vi "HFRR ADV v017 new software.vi"() -> ()   [LabVIEW 2025] (continued)
                n3041 = call <vilib>:"Write Characters To File.vi"("append to file? (new file:F)"=FALSE, "character string"=w3783, "file path (dialog if empty)"=w3788) -> ()  [unwired: 2 in, 1 out]
              }
            }
          }
          frame Enabled {
          }
        }
        n3042 = case shown="True" "OK Button 17" {
          frame False {
          }
          frame True {
            (unwired) 0  # existing file
            w4041 = "Choose a datalog file to open"  # prompt
            n3043 = local write "OK Button 17"(FALSE ("OK Button 17")) -> ()
            n3044 = local read "String"() -> (w4036:string)
            n3045 = String To Path(string=w4036) -> (path=w4037:path)
            n3046 = File Dialog(6:"*.duf" ("pattern"), 7:w4041, 11:w4037) -> (0:w4028:errorcluster, 3:w4047:path)  [unwired: 4 in, 2 out]
            n3047 = Unbundle(w4028) -> ()  [unwired: 3 out]
            n3048 = Open/Create/Replace File "Open File"(file path (use dialog)=w4047) -> (refnum out=w4039:refnum<file>)  [unwired: 5 in, 2 out]
            n3049 = Strip Path(path=w4047) -> (name=w4045:string)  [unwired: 1 out]
            n3050 = Path To String(path=w4047) -> (string=w4030:string)
            n3051 = while {
              tunnel: w4039 -> [w4051]
              i -> [w4048]
              stop <- w4049 continue-if-true
              (unwired) TRUE ("line mode (F)")
              n3052 = Read from Text File "Read File"(file (use dialog)=w4051) -> (text=w4050:string)  [unwired: 3 in, 3 out]
              n3053 = local write "Numeric 16"(w4048) -> ()
              n3054 = String Length(string=w4050) -> (length=w4053:i32)
              n3055 = Greater?(x=w4053, y=1) -> (0:w4049:bool)
            }
            n3056 = local write "String 29"(w4030) -> ()
            n3057 = Search and Replace String(input string=w4030, search string=".duf", replace string=".dgf" ("replace string (\"\")")) -> (result string=→"String Indicator 4":string)  [unwired: 5 in, 3 out]
            n3058 = Match Pattern(string=w4045, regular expression=".dwm") -> (before substring=w4029:string)  [unwired: 1 in, 3 out]
            "String Indicator" <- w4029
            n3059 = Match Pattern(string=w4030, regular expression=".dwm" ("substring (\"\")")) -> (before substring=w4031:string)  [unwired: 1 in, 3 out]
            "String Indicator 3" <- w4031
            n3060 = local write "TITTLE 2"(w4029) -> ()
            n3061 = String To Path(string=w4031) -> (path=w4038:path)
            "path" <- w4038
            n3062 = call <vilib>:"Read Characters From File.vi"("file path (dialog if empty)"=w4038, "start of read offset (chars.:0)"=60 ("start of read offset (chars.: 0)")) -> ("character string"=→"String Indicator 2":string)  [unwired: 4 in, 3 out]
          }
        }
        n3063 = call <vilib>:"Query Available Printers.vi"() -> ("system configured printers"=w3730:string[])  [unwired: 9 in, 2 out]
        "System Configured Printers 2" <- w3730
        n3064 = local read "OK Button 16"() -> (w3727:bool)
        n3065 = case shown="True" "OK Button 16" {
          frame False {
          }
          frame True {
            n3066 = stacked-sequence {
              frame #0 {
                n3067 = local read "Numeric 16"() -> (w4055:i32)
                n3068 = local write "Numeric 10"(w4055) -> ()
              }
              frame #1 {
                n3069 = local read "S.NO"() -> (→"s.NO":string)
                n3070 = local read "String 29"() -> (w4059:string)
                n3071 = String To Path(string=w4059) -> (path=w4058:path)
                n3072 = Open/Create/Replace File "Open File"(file path (use dialog)=w4058) -> (refnum out=w4060:refnum<file>)  [unwired: 5 in, 2 out]
                n3073 = for {
                  N: 16 -> [_]
                  tunnel: w4060 -> [w4067]
                  i -> [w4063]
                  (unwired) TRUE ("line mode (F)")
                  n3074 = Read from Text File "Read File"(file (use dialog)=w4067) -> (text=w4061:string)  [unwired: 3 in, 3 out]
                  n3075 = Match Pattern(string=w4061, regular expression="(") -> (after substring=w4066:string)  [unwired: 1 in, 3 out]
                  n3076 = Match Pattern(string=w4066, regular expression=")") -> (before substring=w4062:string)  [unwired: 1 in, 3 out]
                  n3077 = case shown="1" w4063 {
                    tunnel: w4062 -> [w4068 w4069 _ _ w4070 w4071 w4072 w4074 w4076 w4078 w4080 w4082 w4084 w4086 _]
                    tunnel: w4061 -> [_ _ _ _ _ _ _ _ _ _ _ _ _ _ _]
                    frame 0 {
                      "TITTLE" <- w4068
                    }
                    frame 1 {
                      "Sample ID" <- w4069
                    }
                    frame 2 {
                    }
                    frame 3 {
                    }
                    frame 4 {
                      "Test Date" <- w4070
                    }
                    frame 5 {
                      "Tested by" <- w4071
                    }
                    frame 6 {
                      n3078 = Fract/Exp String To Number(string=w4072) -> (number=→"Humidity before test 2":dbl)  [unwired: 3 in, 1 out]
                    }
                    frame 7 {
                      n3079 = Fract/Exp String To Number(string=w4074) -> (number=→"Temperature before test 2":dbl)  [unwired: 3 in, 1 out]
                    }
                    frame 8 {
                      n3080 = Fract/Exp String To Number(string=w4076) -> (number=→"Humidity after test 2":dbl)  [unwired: 3 in, 1 out]
                    }
                    frame 9 {
                      n3081 = Fract/Exp String To Number(string=w4078) -> (number=→"Temperature after test 2":dbl)  [unwired: 3 in, 1 out]
                    }
                    frame 10 {
                      n3082 = Fract/Exp String To Number(string=w4080) -> (number=→"MWSD 2":dbl)  [unwired: 3 in, 1 out]
                    }
                    frame 11 {
                      n3083 = Fract/Exp String To Number(string=w4082) -> (number=→"AVP 2":dbl)  [unwired: 3 in, 1 out]
                    }
                    frame 12 {
                      n3084 = Fract/Exp String To Number(string=w4084) -> (number=→"HCF 2":dbl)  [unwired: 3 in, 1 out]
                    }
                    frame 13 {
                      n3085 = Fract/Exp String To Number(string=w4086) -> (number=→"WS1.4 2":dbl)  [unwired: 3 in, 1 out]
                    }
                    frame 14, Default {
                    }
                  }
                }
              }
              frame #2 {
              }
            }
            n3086 = local write "OK Button 16"(FALSE ("OK Button 13")) -> ()
          }
        }
        n3087 = Index Array(array=w3730, index="Select Printer 3") -> (element=w3732:string)
        "Selected Printer" <- w3732
        n3088 = case shown="True" w3727 {
          frame False {
          }
          frame True {
            n3089 = flat-sequence {
              frame #0 {
              }
              frame #1 {
                n3090 = Wait (ms)(milliseconds to wait=u32 100) -> ()  [unwired: 1 out]
              }
              frame #2 {
                n3091 = local write "OK Button 16"(FALSE ("Print 3")) -> ()
              }
            }
          }
        }
        n3092 = case shown="True" "Print" {
          tunnel: w3732 -> [_ w4024]
          frame False {
          }
          frame True {
            (unwired) i16 6 ("width (-)")
            (unwired) "TESTED BY : "
            (unwired) "TESTED DATE :"
            (unwired) "SAMPLE ID : "
            (unwired) "SAMPLE DESIGN : "
            w3982 = "\r"
            w3999 = "\r"
            # "add image"
            n3093 = local read "Sample ID"() -> (w3972:string)
            n3094 = local read "Tested by"() -> (w3975:string)
            n3095 = local read "String 34"() -> (w3962:string)
            n3096 = local read "String 45"() -> (w3942:string)
            n3097 = local read "String 35"() -> (w3957:string)
            n3098 = local read "String 37"() -> (w3955:string)
            n3099 = local read "String 32"() -> (w3977:string)
            n3100 = local read "String 36"() -> (w3952:string)
            n3101 = local read "String 31"() -> (w3976:string)
            n3102 = local read "Test Date"() -> (w3973:string)
            n3103 = local read "String 33"() -> (w3978:string)
            n3104 = local read "String 38"() -> (w3948:string)
            n3105 = local read "String 39"() -> (w3945:string)
            n3106 = local write "Print"(FALSE ("Print FF")) -> ()
            n3107 = local read "S 39"() -> (w3960:string)
            n3108 = local read "S 38"() -> (w3967:string)
            n3109 = local read "Temperature before test 2"() -> (w3998:dbl)
            n3110 = local read "Temperature after test 2"() -> (w3988:dbl)
            n3111 = local read "Humidity before test 2"() -> (w4013:dbl)
            n3112 = local read "Humidity after test 2"() -> (w3997:dbl)
            n3113 = local read "MWSD 2"() -> (w4002:dbl)
            n3114 = local read "WS1.4 2"() -> (w3980:dbl)
            n3115 = Concatenate Strings("2)" ("string"), w3962) -> (w3963:string)
            n3116 = Concatenate Strings("3)" ("string"), w3960) -> (w3961:string)
            n3117 = Concatenate Strings("1)" ("string"), w3967) -> (w3966:string)
            n3118 = Concatenate Strings("4)" ("string"), w3957) -> (w3958:string)
            n3119 = Concatenate Strings("5)" ("string"), w3955) -> (w3954:string)
            n3120 = Concatenate Strings("6)" ("string"), w3952) -> (w3951:string)
            n3121 = Concatenate Strings("7)" ("string"), w3948) -> (w3949:string)
            n3122 = Concatenate Strings("8)" ("string"), w3945) -> (w3946:string)
            n3123 = local read "HCF 2"() -> (w3984:dbl)
            n3124 = local read "AVP 2"() -> (w4001:dbl)
            n3125 = local read "s.NO"() -> (w3943:string)
            n3126 = call <vilib>:"New Report.vi"("report type"=enum16{"Standard Report", "HTML"}."Standard Report") -> ("report out"=w4022:refnum<class "NI_report.lvclass">, "error out"=w4021:errorcluster)  [unwired: 13 in]
            n3127 = local read "TITTLE"() -> (w3974:string)
            n3128 = Concatenate Strings(w3999, w3942, w3943, w3999, w3977, w3972, w3999, w3976, w3973, w3999, w3978, w3975, w3999) -> (w3992:string)
            "test by" <- w3992
            n3129 = Number To Fractional String(number=w3998, width (-)=i16 6, precision (6)=i16 2) -> (F-format string=w3987:string)  [unwired: 1 in]
            n3130 = Number To Fractional String(number=w3997, width (-)=i16 6, precision (6)=i16 2) -> (F-format string=w4000:string)  [unwired: 1 in]
            n3131 = Number To Fractional String(number=w4013, width (-)=i16 6, precision (6)=i16 2) -> (F-format string=w4018:string)  [unwired: 1 in]
            n3132 = Number To Fractional String(number=w4002, width (-)=i16 6, precision (6)=i16 2) -> (F-format string=w4004:string)  [unwired: 1 in]
            n3133 = Number To Fractional String(number=w3988, width (-)=i16 6, precision (6)=i16 2) -> (F-format string=w3989:string)  [unwired: 1 in]
            n3134 = Number To Fractional String(number=w4001, width (-)=i16 6, precision (6)=i16 2) -> (F-format string=w4003:string)  [unwired: 1 in]
            n3135 = Number To Fractional String(number=w3984, width (-)=i16 6, precision (6)=i16 2) -> (F-format string=w3983:string)  [unwired: 1 in]
            n3136 = Number To Fractional String(number=w3980, precision (6)=i16 2) -> (F-format string=w3979:string)  [unwired: 2 in]
            n3137 = call-dynamic "Set Report Header Text.vi"("report in"=w4022, "center header text"=w3974, "error in (no error)"=w4021) -> ("report out"=w3993:refnum<class "NI_report.lvclass">, "error out"=w3994:errorcluster)  [unwired: 11 in]
            n3138 = Concatenate Strings(w3982, w3966, w4018, w3982, w3963, w3987, w3982, w3961, w4000, w3982, w3958, w3989, w3982, w3954, w4004, w3982, w3951, w4003, w3982, w3949, w3983, w3982, w3946, w3979) -> (w3970:string)
            "export 2" <- w3970
            n3139 = call-poly <vilib>:"Append Report Text.vi"("report in"=w3993, "text"=w3992, "error in (no error)"=w3994) -> ("report out"=w3996:refnum<class "NI_report.lvclass">, "error out"=w3995:errorcluster)  [unwired: 9 in, 2 out]
            n3140 = local read "test by"() -> (w3969:string)
            n3141 = local read "TITTLE"() -> (w3971:string)
            n3142 = call-poly <vilib>:"Append Report Text.vi"("report in"=w3996, "error in (no error)"=w3995) -> ("report out"=w4017:refnum<class "NI_report.lvclass">, "error out"=w4015:errorcluster)  [unwired: 10 in, 2 out]
            n3143 = Concatenate Strings(w3971, w3970, w3969) -> (→"output":string)
            n3144 = call-poly <vilib>:"Append Report Text.vi"("report in"=w4017, "text"=w3970, "error in (no error)"=w4015) -> ("report out"=w4016:refnum<class "NI_report.lvclass">, "error out"=w4014:errorcluster)  [unwired: 9 in, 2 out]
            n3145 = call-dynamic "Print Report.vi"("report in"=w4016, "printer name (default)"=w4024, "error in (no error)"=w4014) -> ("report out"=w4026:refnum<class "NI_report.lvclass">, "error out"=w4027:errorcluster)  [unwired: 11 in]
            n3146 = call-dynamic "Dispose Report.vi"("report in"=w4026, "error in (no error)"=w4027) -> ()  [unwired: 13 in, 1 out]
          }
        }
        n3147 = case shown="True" "Print 2" {
          frame False {
          }
          frame True {
            n3148 = flat-sequence {
              frame #0 {
                n3149 = local read "s.NO"() -> (→"s.NO 2":string)
                n3150 = Wait (ms)(milliseconds to wait=u32 20) -> ()  [unwired: 1 out]
                n3151 = local read "Sample ID  3"() -> (→"Sample ID  6":string)
                n3152 = local read "Sample ID  4"() -> (→"Sample ID  7":string)
                n3153 = local read "Sample ID"() -> (→"Sample ID  2":string)
                n3154 = local read "Tested by"() -> (→"Tested by 2":string)
                n3155 = local read "Test Date"() -> (→"Test Date 2":string)
                n3156 = local read "Humidity after test 3"() -> (→"Humidity after test 4":dbl)
                n3157 = local read "Ref A Test Date :"() -> (→"TITTLE 4":string)
                n3158 = local read "Temperature before test 3"() -> (w3849:dbl)
                n3159 = local read "Temperature before test 3"() -> (→"Temperature after test 5":dbl)
                n3160 = local read "Temperature after test 3"() -> (→"Temperature after test 4":dbl)
                n3161 = local read "Humidity before test 3"() -> (→"Humidity before test 4":dbl)
                n3162 = local write "Temperature before test 3"(w3849) -> ()
                n3163 = local read "image data"() -> (w3840:T16)
                n3164 = String To Path(string="C:\\LAB-IQ\\im\\Temp_resized.jpg") -> (path=w3841:path)
                "path 2" <- w3841
                n3165 = call <vilib>:"Write JPEG File.vi"("image data"=w3840, "path to JPEG file"=w3841) -> ()  [unwired: 8 in, 2 out]
                "Ref A Test Date :" <- "Ref A Test Date :"
                "Ref B Test Date :" <- "Ref B Test Date :"
                "Ref B Scar Value :" <- "Ref B Scar Value :"
                "Ref A Scar Value :" <- "Ref A Scar Value :"
              }
              frame #1 {
                (unwired) HTML_Report_Image_Alignment."MIDDLE" ("alignment (default)")
                w3877 = u16 0 items=["portrait", "landscape"] ("orientation (portrait)")
                (unwired) HTML_Report_Image_Alignment."ABSMIDDLE" ("alignment (default)")
                (unwired) "TESTED BY : "
                (unwired) "TESTED DATE :"
                (unwired) "SAMPLE ID : "
                (unwired) "SAMPLE DESIGN : "
                w3910 = "\r"
                # "add image"
                n3166 = Wait (ms)(milliseconds to wait=u32 20) -> ()  [unwired: 1 out]
                n3167 = local read "Sample ID  2"() -> (w3903:string)
                n3168 = local read "Wear Scar X"() -> (w3875:dbl)
                "Length ( microns ) 2" <- w3875
                n3169 = local read "Wear Scar Y"() -> (w3874:dbl)
                "Wear Scar Y ( microns ) :" <- w3874
                n3170 = local read "Test Date 2"() -> (w3904:string)
                n3171 = local read "Tested by 2"() -> (w3905:string)
                n3172 = local read "String 46"() -> (w3901:string)
                n3173 = local read "String 48"() -> (w3907:string)
                n3174 = local read "String 47"() -> (w3906:string)
                n3175 = local read "String 49"() -> (w3908:string)
                n3176 = local read "String 10"() -> (w3861:string)
                n3177 = local read "s.NO 2"() -> (w3902:string)
                n3178 = Add(x=w3875, y=w3874) -> (x+y=w3873:dbl)
                n3179 = call <vilib>:"New Report.vi"("report type"=enum16{"Standard Report", "HTML"}."HTML") -> ("report out"=w3881:refnum<class "NI_report.lvclass">, "error out"=w3879:errorcluster)  [unwired: 13 in]
                n3180 = Concatenate Strings(w3910, w3901, w3902, w3910, w3907, w3903, w3910, w3906, w3904, w3910, w3908, w3905, w3910) -> (→"test by 2":string)
                n3181 = Concatenate Strings("C:\\LAB-IQ\\Data\\" ("string"), w3861, ".jpg" ("string")) -> ()  [unwired: 1 out]
                n3182 = Divide(x=w3873, y=2.0) -> (x/y=→"Mean Wear ( microns) :":dbl)
                n3183 = call-dynamic "Set Report Orientation.vi"("report in"=w3881, "orientation (portrait)"=w3877, "error in (no error)"=w3879) -> ("report out"=w3880:refnum<class "NI_report.lvclass">, "error out"=w3878:errorcluster)  [unwired: 11 in]
                n3184 = for {
                  N: 5 -> [_]
                  tunnel: w3880 -> [w3931]
                  tunnel: [w3930] -> w3859
                  tunnel: w3878 -> [w3929]
                  tunnel: [w3928] -> w3858
                  n3185 = call-dynamic "Set Report Tab Width.vi"("report in"=w3931, "error in (no error)"=w3929) -> ("report out"=w3930:refnum<class "NI_report.lvclass">, "error out"=w3928:errorcluster)  [unwired: 12 in]
                }
                n3186 = local read "TITTLE"() -> (w3876:string)
                n3187 = call-dynamic "Set Report Header Text.vi"("report in"=w3859, "center header text"=w3876, "error in (no error)"=w3858) -> ("report out"=w3897:refnum<class "NI_report.lvclass">, "error out"=w3896:errorcluster)  [unwired: 11 in]
                n3188 = for {
                  N: 1 -> [_]
                  tunnel: [w3935] -> w3883
                  tunnel: [w3934] -> w3882
                  tunnel: w3897 -> [w3933]
                  tunnel: w3896 -> [w3932]
                  n3189 = call-dynamic "New Report Line.vi"("report in"=w3933, "error in (no error)"=w3932) -> ("report out"=w3935:refnum<class "NI_report.lvclass">, "error out"=w3934:errorcluster)  [unwired: 12 in]
                }
                n3190 = for {
                  N: 2 -> [_]
                  tunnel: [w3927] -> w3889
                  tunnel: [w3926] -> w3888
                  tunnel: w3883 -> [w3925]
                  tunnel: w3882 -> [w3924]
                  n3191 = call-dynamic "New Report Line.vi"("report in"=w3925, "error in (no error)"=w3924) -> ("report out"=w3927:refnum<class "NI_report.lvclass">, "error out"=w3926:errorcluster)  [unwired: 12 in]
                }
                n3192 = for {
                  N: 25 -> [_]
                  tunnel: w3889 -> [w3923]
                  tunnel: w3888 -> [w3921]
                  tunnel: [w3922] -> w3892
                  tunnel: [w3920] -> w3891
                  n3193 = call-dynamic "Set Report Tab Width.vi"("report in"=w3923, "error in (no error)"=w3921) -> ("report out"=w3922:refnum<class "NI_report.lvclass">, "error out"=w3920:errorcluster)  [unwired: 12 in]
                }
                n3194 = control-ref of="Tab Control 9"() -> (w3887:refnum<vi>)
                n3195 = call-dynamic "Append Control Image to Report.vi"("report in"=w3892, "alignment (default)"=HTML_Report_Image_Alignment."ABSMIDDLE", "ctrl reference"=w3887, "error in (no error)"=w3891) -> ("report out"=w3886:refnum<class "NI_report.lvclass">, "error out"=w3885:errorcluster)  [unwired: 8 in, 2 out]
                n3196 = for {
                  N: 3 -> [_]
                  tunnel: [w3919] -> w3870
                  tunnel: [w3918] -> w3869
                  tunnel: w3886 -> [w3917]
                  tunnel: w3885 -> [w3916]
                  n3197 = call-dynamic "New Report Line.vi"("report in"=w3917, "error in (no error)"=w3916) -> ("report out"=w3919:refnum<class "NI_report.lvclass">, "error out"=w3918:errorcluster)  [unwired: 12 in]
                }
                n3198 = for {
                  N: 100 -> [_]
                  tunnel: w3870 -> [w3915]
                  tunnel: w3869 -> [w3913]
                  tunnel: [w3914] -> w3866
                  tunnel: [w3912] -> w3864
                  n3199 = call-dynamic "Set Report Tab Width.vi"("report in"=w3915, "error in (no error)"=w3913) -> ("report out"=w3914:refnum<class "NI_report.lvclass">, "error out"=w3912:errorcluster)  [unwired: 12 in]
                }
                n3200 = String To Path(string="C:\\LAB-IQ\\im\\Temp_resized.jpg") -> (path=w3856:path)
                n3201 = call-poly <vilib>:"Append Image to Report.vi"("report in"=w3866, "path or URL of image"=w3856, "error in (no error)"=w3864) -> ("report out"=w3865:refnum<class "NI_report.lvclass">, "error out"=w3863:errorcluster)  [unwired: 9 in, 2 out]
                n3202 = call-poly <vilib>:"Open HTML Report in Browser.vi"("report in"=w3865, "error in (no error)"=w3863) -> ("report out"=w3900:refnum<class "NI_report.lvclass">, "error out"=w3899:errorcluster)  [unwired: 11 in, 1 out]
                n3203 = call-dynamic "Dispose Report.vi"("report in"=w3900, "error in (no error)"=w3899) -> ()  [unwired: 13 in, 1 out]
              }
              frame #2 {
              }
              frame #3 {
                n3204 = disable-structure shown="Disabled" {
                  frame Disabled {
                    n3205 = local read "String 10"() -> (w3940:string)
                    n3206 = Concatenate Strings("C:\\LAB-IQ-NXT\\Data\\" ("string"), w3940, ".jpg" ("string")) -> (w3938:string)
                    n3207 = String To Path(string=w3938) -> (path=w3937:path)
                    n3208 = Delete(path (use dialog)=w3937) -> ()  [unwired: 4 in, 3 out]
                  }
                  frame Enabled {
                  }
                }
                n3209 = local write "Print 2"(FALSE ("Print")) -> ()
              }
            }
          }
        }
      }
    }
    n3210 = property on="SetTemp" class="DigNum (strict)"("Disabled"=w1876) -> ()  [unwired: 2 in, 2 out]
    n3211 = Multiply(x=w1866, y=w1868) -> (x*y=w1867:dbl)
    n3212 = local read "MWSD"() -> (w1865:dbl)
    n3213 = Add(x=w1867, y=w1865) -> (x+y=→"WS1.4":dbl)
    n3214 = Wait (ms)(milliseconds to wait=u32 50) -> ()  [unwired: 1 out]
    n3215 = Wait (ms)(milliseconds to wait=u32 50) -> ()  [unwired: 1 out]
    n3216 = local read "Quit"() -> (w1864:bool)
  }
  n3217 = VISA Close(VISA resource name=w53, error in (no error)=w52) -> (error out=w50:errorcluster)
  n3218 = call <vilib>:"Clear Errors.vi"("error in (no error)"=w50) -> ()  [unwired: 5 in, 2 out]
  n3219 = VISA Close(VISA resource name=w38, error in (no error)=w37) -> ()  [unwired: 1 out]
  n3220 = while {
    tunnel: [w4101] -> w47
    shift-right: [w4094] -> _
    shift-left: 0.0 -> [w4097]
    shift-right: [w4093] -> _
    shift-left: 0.0 -> [w4096]
    shift-right: [w4092] -> _
    shift-left: 400.0 ("vc_cmd") -> [w4095]
    stop <- w4101 stop-if-true
    # "PID LOGIC"
    n3221 = local read "RUN"() -> (w4099:bool)
    n3222 = local read "Auto Start Temp"() -> (w4088:bool)
    n3223 = local read "Auto Start Test"() -> (w4098:bool)
    n3224 = local read "START TEMP"() -> (w4090:bool)
    n3225 = And(x=w4088, y=w4098) -> (x .and. y?=w4089:bool)
    n3226 = Or(x=w4099, y=w4089) -> (x .or. y?=w4100:bool)
    n3227 = And(x=w4100, y=w4090) -> (x .and. y?=w4091:bool)
    n3228 = Wait (ms)(milliseconds to wait=u32 20) -> ()  [unwired: 1 out]
    n3229 = case shown="True" w4091 {
      tunnel: [400.0 ("out_vc_cmd") w4121] -> w4092
      tunnel: [w4104 w4123] -> w4093
      tunnel: [w4104 w4122] -> w4094
      tunnel: w4097 -> [_ w4112]
      tunnel: w4096 -> [_ w4111]
      tunnel: w4095 -> [_ w4110]
      frame False {
        w4104 = 0.0 ("error_out")
      }
      frame True {
        n3230 = local read "Set Strk"() -> (w4107:dbl)
        n3231 = local read "LVDT STROKE"() -> (w4105:dbl)
        n3232 = Add(x=w4107, y="Add up Stroke") -> (x+y=w4108:dbl)
        n3233 = formula code="// Zero-Hardcode Explicit Positional-Form PID Engine\n// Inputs: target_stroke, measured_stroke, dt, prev_error, integral_accumulator_in, prev_vc_cmd\n//         kp, ki, kd, max_step_change, max_amplitude, min_amplitude, startup_cmd\n// Outputs: vc_cmd, error_out, out_error, integral_accumulator_out, out_vc_cmd\n\n// 1. Calculate Tracking Error\nfloat current_error = target_stroke - measured_stroke;\nerror_out = current_error;\n\n// 2. Compute Proportional Term\nfloat p_term = kp * current_error;\n\n// 3. Compute Derivative Term\nfloat d_term = 0.0;\nif (dt > 0.0) {\n    d_term = kd * ((current_error - prev_error) / dt);\n}\n\n// 4. Update and Accumulate Integral Term\nfloat current_integral = integral_accumulator_in + (current_error * dt);\nfloat i_term = ki * current_integral;\n\n// 5. Calculate Ideal Target Command\nfloat ideal_command = startup_cmd + p_term + i_term + d_term;\n\n// 6. Anti-Windup Protection (Back-calculation method)\nif (ideal_command > max_amplitude) {\n    float excess = ideal_command - max_amplitude;\n    if (ki > 0.0) {\n        current_integral -= excess / ki;\n    }\n    ideal_command = max_amplitude;\n} else if (ideal_command < min_amplitude) {\n    float excess = ideal_command - min_amplitude;\n    if (ki > 0.0) {\n        current_integral -= excess / ki;\n    }\n    ideal_command = min_amplitude;\n}\n\n// 7. Apply Loop Rate Limiting (Protects voice coil from large voltage steps)\nfloat raw_adjustment = ideal_command - prev_vc_cmd;\n\nif (raw_adjustment > max_step_change) {\n    raw_adjustment = max_step_change;\n} else if (raw_adjustment < -max_step_change) {\n    raw_adjustment = -max_step_change;\n}\n\nfloat next_vc_cmd = prev_vc_cmd + raw_adjustment;\n\n// Final Output Safety Safeguard Clamping\nif (next_vc_cmd > max_amplitude) {\n    next_vc_cmd = max_amplitude;\n} else if (next_vc_cmd < min_amplitude) {\n    next_vc_cmd = min_amplitude;\n}\n\n// 8. Map to Shift Registers for memory persistence\nvc_cmd = next_vc_cmd;\nout_error = current_error;                     \nintegral_accumulator_out = current_integral;  \nout_vc_cmd = next_vc_cmd;"("target_stroke"=w4108, "measured_stroke"=w4105, "dt"="dt", "integral_accumulator_in"=w4111, "prev_error"=w4112, "prev_vc_cmd"=w4110, "kp"="kp", "ki"="ki", "kd"="kd", "max_step_change"="max_step_change", "max_amplitude"="max_amplitude", "min_amplitude"="min_amplitude", "startup_cmd"="startup_cmd") -> ("vc_cmd"=w4127:dbl, "out_error"=w4122:dbl, "integral_accumulator_out"=w4123:dbl, "out_vc_cmd"=w4121:dbl)  [unwired: 1 out]
        "output Vpp" <- w4127
        n3234 = Number To Fractional String(number=w4127, precision (6)=i16 1) -> (F-format string=w4125:string)  [unwired: 2 in]
        n3235 = Concatenate Strings("DAC;" ("string"), w4125) -> (w4109:string)
        n3236 = local write "Command"(w4109) -> ()
        "prev_error" <- w4112
        "integral_accumulator_in" <- w4111
        "prev_vc_cmd" <- w4110
      }
    }
    n3237 = local read "Quit"() -> (w4101:bool)
  }
  n3238 = Or(x=w43, y=w42) -> (x .or. y?=w44:bool)
  n3239 = Or(x=w40, y=w44) -> (x .or. y?=w49:bool)
  n3240 = control-ref of="new picture"() -> ()  [unwired: 1 out]
  n3241 = Or(x=w55, y=w49) -> (x .or. y?=w46:bool)
  n3242 = Or(x=w46, y=w47) -> (x .or. y?=w41:bool)
  n3243 = while {
    tunnel: [w4128] -> w54
    i -> [w4135]
    stop <- w4128 stop-if-true
    n3244 = local read "Quit"() -> (w4128:bool)
    n3245 = Equal To 0?(x=w4135) -> (x = 0?=w4133:bool)
    n3246 = call "Elapsed Time3"("Time Target (s)"=45.0, "Auto Reset"=TRUE) -> ("Time has Elapsed"=w4132:bool)  [unwired: 10 in, 7 out]
    n3247 = Wait (ms)(milliseconds to wait=u32 50) -> ()  [unwired: 1 out]
    n3248 = Or(x=w4132, y=w4133) -> (x .or. y?=w4134:bool)
    n3249 = case shown="True" w4134 {
      frame False {
      }
      frame True {
        n3250 = call <vilib>:"System Exec.vi"("run minimized? (F)"=TRUE, "error in (no error)"="error in (no error)", "command line"="powercfg.exe -change -monitor-timeout-ac 0") -> ("error out"=w4146:errorcluster)  [unwired: 5 in, 3 out]
        n3251 = call <vilib>:"System Exec.vi"("run minimized? (F)"=TRUE, "error in (no error)"=w4146, "command line"="powercfg.exe -change -disk-timeout-ac 0") -> ("error out"=w4145:errorcluster)  [unwired: 5 in, 3 out]
        n3252 = call <vilib>:"System Exec.vi"("run minimized? (F)"=TRUE, "error in (no error)"=w4145, "command line"="powercfg.exe -change -standby-timeout-ac 0") -> ("error out"=w4144:errorcluster)  [unwired: 5 in, 3 out]
        n3253 = call <vilib>:"System Exec.vi"("run minimized? (F)"=TRUE, "error in (no error)"=w4144, "command line"="powercfg.exe -change -hibernate-timeout-ac 0") -> ("error out"=w4143:errorcluster)  [unwired: 5 in, 3 out]
        n3254 = call <vilib>:"Simple Error Handler.vi"("error in (no error)"=w4143) -> ("error out"=w4149:errorcluster)  [unwired: 4 in, 4 out]
        n3255 = call <vilib>:"Clear Errors.vi"("error in (no error)"=w4149) -> ("error out"=→"error out":errorcluster)  [unwired: 5 in, 1 out]
      }
    }
  }
  n3256 = Compound Arithmetic op=OR(w57, w41, w54) -> (w56:bool)
  n3257 = flat-sequence {
    tunnel: w56 -> [_]
    tunnel: [w4151] -> w19
    tunnel: w19 -> [_]
    frame #0 {
      n3258 = call "CLOSE CONNECTION.vi"() -> ("error out"=w4151:errorcluster)  [unwired: 11 in]
    }
    frame #1 {
      n3259 = Quit LabVIEW(quit? (T)=TRUE) -> ()
      n3260 = local write "Quit"(FALSE ("EXIT")) -> ()
    }
  }
  n3261 = property on="Heater Button" class="Bool (strict)"("Visible"=TRUE) -> ()  [unwired: 2 in, 2 out]
  n3262 = disable-structure shown="Disabled" {
    disable-tunnel: _ -> [w4157 _]
    disable-tunnel: _ -> [w4154 _]
    disable-tunnel: _ -> [w4155 _]
    frame Disabled {
      n3263 = disable-structure shown="Disabled" {
        disable-tunnel: [w4164 _] -> w4156
        frame Disabled {
          n3264 = while {
            shift-right: [w4206] -> w4162
            shift-left: errorcluster {"status"=TRUE, "code"=0, "source"="Init"} ("error out") -> [w4171]
            shift-right: [w4205] -> w4161
            shift-left: _ -> [w4172]
            shift-right: [w4204] -> _
            shift-left: "" -> [w4203]
            tunnel: [w4165] -> w4164
            shift-right: ["Set Rh"] -> _
            shift-left: 0.0 ("Set Rh") -> [w4197]
            tunnel: [w4174] -> _
            i -> [w4174]
            stop <- w4165 stop-if-true
            n3265 = flat-sequence {
              tunnel: w4171 -> [w4209]
              tunnel: [w4209] -> w4170
              frame #0 {
                n3266 = Wait (ms)(milliseconds to wait=u32 200) -> ()  [unwired: 1 out]
              }
            }
            n3267 = local read "Com Port 3"() -> (w4173:refnum<visa-resource-name>)
            n3268 = local read "Humidity Str Rec"() -> (w4175:string)
            n3269 = Not Equal?(x="Set Rh", y=w4197) -> (x != y?=w4202:bool)
            n3270 = Number To Decimal String(number="Set Rh") -> (decimal integer string=w4200:string)  [unwired: 1 in]
            n3271 = Not Equal?(x=w4173, y=w4172) -> (x != y?=w4168:bool)
            n3272 = Concatenate Strings("#setPoint00" ("string"), w4200) -> (w4201:string)
            n3273 = case shown="False" w4202 {
              tunnel: w4201 -> [_ w4221]
              frame False {
                n3274 = local read "Humidity"() -> (w4218:bool)
                n3275 = case shown="True" w4218 {
                  frame False {
                    n3276 = local write "Humidity Str Send"("stop" ("Humidity Str Send")) -> ()
                  }
                  frame True {
                    n3277 = local write "Humidity Str Send"("start" ("Humidity Str Send")) -> ()
                  }
                }
              }
              frame True {
                n3278 = local write "Humidity Str Send"(w4221) -> ()
              }
            }
            n3279 = Or(x=w4168) -> (y=w4166:bool, x .or. y?=w4167:bool)
            n3280 = String Subset(string=w4175, offset (0)=7) -> (substring=w4190:string)  [unwired: 1 in]
            n3281 = Match Pattern(string=w4175, regular expression="?") -> (offset past match=w4193:i32)  [unwired: 1 in, 3 out]
            n3282 = Match Pattern(string=w4175, regular expression="v") -> (offset past match=w4196:i32)  [unwired: 1 in, 3 out]
            n3283 = case shown="True" w4167 {
              tunnel: w4170 -> [w4207 _]
              tunnel: [w4207 errorcluster {"status"=TRUE, "code"=0, "source"="Init"} ("error out")] -> w4169
              frame False {
              }
              frame True {
              }
            }
            n3284 = Equal?(x=w4193, y=-1) -> (x = y?=w4177:bool)
            n3285 = Match Pattern(string=w4190, regular expression="g") -> (after substring=w4191:string, offset past match=w4182:i32)  [unwired: 1 in, 2 out]
            n3286 = Match Pattern(string=w4190, regular expression="y") -> (after substring=w4189:string, offset past match=w4183:i32)  [unwired: 1 in, 2 out]
            n3287 = Greater?(x=w4183, y=w4182) -> (0:w4188:bool)
            n3288 = Greater Or Equal To 0?(x=w4183) -> (x >= 0?=w4180:bool)
            n3289 = Greater Or Equal To 0?(x=w4182) -> (x >= 0?=w4181:bool)
            n3290 = Or(x=w4180, y=w4181) -> (x .or. y?=w4179:bool)
            n3291 = Greater Or Equal To 0?(x=w4196) -> (x >= 0?=w4178:bool)
            n3292 = Select(t=w4189, s=w4188, f=w4191) -> (s? t:f=w4184:string)
            n3293 = case shown="Error" w4169 {
              selector: w4169 -> [w4234 w4280]
              tunnel: [w4232 w4273] -> w4206
              tunnel: w4172 -> [w4235 w4279]
              tunnel: [w4233 w4282] -> w4205
              tunnel: w4203 -> [w4222 w4281]
              tunnel: [w4229 w4281] -> w4204
              frame No Error {
                n3294 = call "Elapsed Time7"() -> ("Time has Elapsed"=w4228:bool)  [unwired: 12 in, 7 out]
                n3295 = Not Equal?(x="Humidity Str Send", y=w4222) -> (x != y?=w4224:bool)
                n3296 = Or(x=w4224, y=w4228) -> (x .or. y?=w4227:bool)
                n3297 = Select(t="Humidity Str Send", s=w4224, f="vals" ("regular expression")) -> (s? t:f=w4223:string)
                n3298 = Or(x=w4227, y="Send") -> (x .or. y?=w4231:bool)
                n3299 = case shown="True" w4231 {
                  tunnel: [w4238 w4243] -> w4232
                  tunnel: w4235 -> [w4237 w4251]
                  tunnel: w4234 -> [w4238 w4250]
                  tunnel: [w4237 w4244] -> w4233
                  tunnel: w4223 -> [_ w4249]
                  tunnel: [w4236 w4240] -> w4229
                  tunnel: "Humidity Str Send" -> [_ w4241]
                  tunnel: w4224 -> [_ w4242]
                  tunnel: w4222 -> [w4236 w4239]
                  frame False {
                  }
                  frame True {
                    n3300 = flat-sequence {
                      tunnel: w4251 -> [w4259]
                      tunnel: w4250 -> [w4258]
                      tunnel: w4249 -> [w4255]
                      tunnel: [w4257] -> w4248
                      tunnel: [w4256] -> w4247
                      tunnel: w4248 -> [w4262]
                      tunnel: w4247 -> [w4261]
                      tunnel: [w4262] -> w4246
                      tunnel: [w4261] -> w4245
                      tunnel: w4246 -> [w4269]
                      tunnel: w4245 -> [w4268]
                      tunnel: [w4267] -> w4244
                      tunnel: [w4266] -> w4243
                      frame #0 {
                        n3301 = local write "Ser Led"(TRUE ("Boolean 4")) -> ()
                        n3302 = Concatenate Strings(w4255, "\r") -> (w4254:string)
                        n3303 = VISA Write(VISA resource name=w4259, write buffer=w4254, error in (no error)=w4258) -> (VISA resource name out=w4257:refnum<visa-resource-name>, error out=w4256:errorcluster)  [unwired: 1 out]
                      }
                      frame #1 {
                        n3304 = Wait (ms)(milliseconds to wait="wait") -> ()  [unwired: 1 out]
                      }
                      frame #2 {
                        w4264 = FALSE ("Send")
                        n3305 = property class="Instr"(reference=w4269, error in=w4268) -> (reference out=w4270:refnum<visa-resource-name>, error out=w4271:errorcluster, "Serial Settings:Number of Bytes at Serial Port"=w4263:u32)
                        n3306 = local write "Send"(w4264) -> ()
                        n3307 = local write "Ser Led"(w4264) -> ()
                        n3308 = VISA Read(VISA resource name=w4270, byte count=w4263, error in (no error)=w4271) -> (VISA resource name out=w4267:refnum<visa-resource-name>, read buffer=→"Humidity Str Rec":string, error out=w4266:errorcluster)  [unwired: 1 out]
                      }
                    }
                    n3309 = Select(t=w4241, s=w4242, f=w4239) -> (s? t:f=w4240:string)
                  }
                }
              }
              frame Error {
                w4287 = u16 0 items=["None"=0, "XON/XOFF"=1, "RTS/CTS"=2, "DTR/DSR"=4] ("flow control")
                w4283 = u16 0 items=["None", "Odd", "Even", "Mark", "Space"] ("parity")
                w4286 = u16 10 items=["1.0"=10, "1.5"=15, "2.0"=20] ("stop bits")
                n3310 = VISA Close(VISA resource name=w4279, error in (no error)=w4280) -> (error out=w4278:errorcluster)
                n3311 = local write "humid"("" ("humid")) -> ()
                n3312 = local write "Humidity Str Rec"("" ("Humidity Str Rec")) -> ()
                n3313 = call <vilib>:"Clear Errors.vi"("error in (no error)"=w4278) -> ("error out"=w4277:errorcluster)  [unwired: 5 in, 1 out]
                n3314 = local read "Com Port 3"() -> (w4276:refnum<visa-resource-name>)
                n3315 = call-poly "VISA Configure Serial Port"("VISA resource name"=w4276, "timeout (10sec)"=u32 1000, "termination char\n(0xA = '\\n' = LF)"=u8 10 ("termination char\n(0xA = '\\n' = LF)"), "Enable Termination\nChar (T)"=FALSE ("Enable Termination Char (T)"), "data bits (8)"=u16 8 ("data bits"), "parity (0:none)"=w4283, "error in (no error)"=w4277, "stop bits (10: 1 bit)"=w4286, "flow control (0:none)"=w4287) -> ("VISA resource name out"=w4282:refnum<visa-resource-name>, "baud rate (9600)"=w4274:u32, "error out"=w4273:errorcluster)  [unwired: 4 in]
              }
            }
            n3316 = Compound Arithmetic op=AND(w4178, w4177, w4179) -> (w4176:bool)
            n3317 = case shown="True" w4176 {
              tunnel: w4175 -> [_ _]
              tunnel: w4184 -> [_ w4214]
              frame False {
              }
              frame True {
                w4212 = " " ("regular expression")
                n3318 = Match Pattern(string=w4214, regular expression=" ") -> (after substring=w4216:string)  [unwired: 1 in, 3 out]
                n3319 = Match Pattern(string=w4216, regular expression=w4212) -> (before substring=→"humid":string, after substring=w4213:string)  [unwired: 1 in, 2 out]
                n3320 = Match Pattern(string=w4213, regular expression=w4212) -> (before substring=→"temp_@Rh sensor":string)  [unwired: 1 in, 3 out]
              }
            }
            n3321 = local read "Quit"() -> (w4165:bool)
          }
          n3322 = VISA Close(VISA resource name=w4161, error in (no error)=w4162) -> (error out=w4158:errorcluster)
          n3323 = call <vilib>:"Clear Errors.vi"("error in (no error)"=w4158) -> ()  [unwired: 5 in, 2 out]
        }
        frame Enabled {
        }
      }
    }
    frame Enabled {
    }
  }
  n3324 = while {
    tunnel: [w4294] -> _
    i -> [w4294]
    stop <- w4290 stop-if-true
    # "Langauage selection"
    n3325 = Equal?(x="Lan flag", y=22.0) -> ()  [unwired: 1 out]
    n3326 = disable-structure shown="Disabled" {
      frame Disabled {
        n3327 = stacked-sequence {
          frame #0 {
            n3328 = case shown="\"Russian\"" "Language Selection" {
              tunnel: [0 1] -> w4296
              frame "English", Default {
              }
              frame "Russian" {
              }
            }
            n3329 = for {
              N: 130 -> [_]
              tunnel: "Table" -> [w4305]
              tunnel: w4296 -> [w4304]
              i -> [w4303]
              n3330 = Index Array(array=w4305, index (row)=w4303, index (col)=w4304) -> (element=w4302:string)
              n3331 = case shown="123" w4303 {
                tunnel: w4302 -> [w4306 w4307 _ w4308 w4309 w4310 w4311 w4312 w4313 w4314 w4315 w4316 w4317 w4318 w4319 w4320 w4321 w4322 w4323 w4324 w4325 w4326 w4327 w4328 w4329 w4330 w4331 w4332 w4333 _ _ w4334 w4335 w4336 w4337 w4338 w4339 w4348 w4355 w4362 w4369 w4373 w4376 w4379 w4381 w4383 w4384 w4385 w4386 w4387 w4388 w4389 w4390 w4391 w4392 w4393 w4394 w4395 w4396 w4397 w4398 w4399 w4400 w4401 w4402 w4403 w4404 w4405 w4406 w4407 w4408 w4409 w4410 w4411 w4412 w4413 w4414 w4415 w4416 w4417 w4418 w4419 w4420 w4421 w4422 w4423 w4424 w4425 w4426 w4427 w4428 w4429 w4430 w4431 w4432 w4433 w4434 w4435 w4436 w4437 w4438 w4439 w4440 w4441 w4442 _ w4443 w4444 w4445 w4446 w4447 w4448 w4449 w4450 w4451 w4452 w4453 w4454 w4455 _ w4456 w4457 w4458 w4459 w4460 w4461 _]
                frame 0 {
                  n3332 = local write "S"(w4306) -> ()
                }
                frame 1 {
                  n3333 = local write "S 2"(w4307) -> ()
                }
                frame 2 {
                }
                frame 3 {
                  n3334 = local write "S 4"(w4308) -> ()
                }
                frame 4 {
                  n3335 = property on="FILE" class="Str"("Caption.Text"=w4309) -> ()  [unwired: 2 in, 2 out]
                }
                frame 5 {
                  n3336 = property on="Fuel Discription :" class="Str"("Caption.Text"=w4310) -> ()  [unwired: 2 in, 2 out]
                }
                frame 6 {
                  n3337 = property on="Remarks :" class="Str"("Caption.Text"=w4311) -> ()  [unwired: 2 in, 2 out]
                }
                frame 7 {
                  n3338 = property on="Save & Continue" class="Bool (strict)"("Boolean Text.Text"=w4312) -> ()  [unwired: 2 in, 2 out]
                }
                frame 8 {
                }
                frame 9 {
                  n3339 = property on="Set Hz" class="DigNum (strict)"("Caption.Text"=w4314) -> ()  [unwired: 2 in, 2 out]
                }
                frame 10 {
                  "String 3" <- w4315
                }
                frame 11 {
                  n3340 = property on="NORMAL LOAD" class="DigNum (strict)"("Caption.Text"=w4316) -> ()  [unwired: 2 in, 2 out]
                }
                frame 12 {
                  "String 5" <- w4317
                }
                frame 13 {
                  n3341 = property on="Set Temp" class="DigNum (strict)"("Caption.Text"=w4318) -> ()  [unwired: 2 in, 2 out]
                }
                frame 14 {
                  n3342 = local write "S 15"(w4319) -> ()
                }
                frame 15 {
                  n3343 = property on="Set Rh" class="DigNum (strict)"("Caption.Text"=w4320) -> ()  [unwired: 2 in, 2 out]
                }
                frame 16 {
                  "String 13" <- w4321
                  "String 26" <- w4321
                }
                frame 17 {
                  n3344 = local write "S 18"(w4322) -> ()
                }
                frame 18 {
                  "String 17" <- w4323
                }
                frame 19 {
                  n3345 = property on="test time" class="DigNum (strict)"("Caption.Text"=w4324) -> ()  [unwired: 2 in, 2 out]
                }
                frame 20 {
                  "String 18" <- w4325
                  "String 22" <- w4325
                }
                frame 21 {
                  n3346 = property on="Elapsed time" class="DigNum (strict)"("Caption.Text"=w4326) -> ()  [unwired: 2 in, 2 out]
                }
                frame 22 {
                  n3347 = property on="Samplingtime 2" class="DigNum (strict)"("Caption.Text"=w4327) -> ()  [unwired: 2 in, 2 out]
                }
                frame 23 {
                  "String 21" <- w4328
                }
                frame 24 {
                  n3348 = property on="Countdown" class="DigNum (strict)"("Caption.Text"=w4329) -> ()  [unwired: 2 in, 2 out]
                }
                frame 25 {
                  n3349 = property on="Countdown 2" class="DigNum (strict)"("Caption.Text"=w4330) -> ()  [unwired: 2 in, 2 out]
                }
                frame 26 {
                  n3350 = property on="Engage" class="Bool (strict)"("Boolean Text.Text"=w4331) -> ()  [unwired: 2 in, 2 out]
                }
                frame 27 {
                  n3351 = property on="Boolean  4" class="Bool (strict)"("Boolean Text.Text"=w4332) -> ()  [unwired: 2 in, 2 out]
                }
                frame 28 {
                  n3352 = property on="Test \nStatus" class="Bool (strict)"("Boolean Text.Text"=w4333) -> ()  [unwired: 2 in, 2 out]
                }
                frame 29 {
                }
                frame 30 {
                }
                frame 31 {
                }
                frame 32 {
                  n3353 = property on="RSTCOF" class="Bool"("Boolean Text.Text"=w4335) -> ()  [unwired: 2 in, 2 out]
                  n3354 = property on="RST FF" class="Bool"("Boolean Text.Text"=w4335) -> ()  [unwired: 2 in, 2 out]
                  n3355 = property on="RST TEMP" class="Bool"("Boolean Text.Text"=w4335) -> ()  [unwired: 2 in, 2 out]
                  n3356 = property on="RSTV1 3" class="Bool"("Boolean Text.Text"=w4335) -> ()  [unwired: 2 in, 2 out]
                  n3357 = property on="rstv2" class="Bool"("Boolean Text.Text"=w4335) -> ()  [unwired: 2 in, 2 out]
                  n3358 = property on="RSTV1 2" class="Bool"("Boolean Text.Text"=w4335) -> ()  [unwired: 2 in, 2 out]
                  n3359 = property on="RST CP" class="Bool"("Boolean Text.Text"=w4335) -> ()  [unwired: 2 in, 2 out]
                }
                frame 33 {
                  "S 61" <- w4336
                }
                frame 34 {
                  "String 23" <- w4337
                }
                frame 35 {
                  n3360 = property on="Rh Before" class="DigNum (strict)"("Caption.Text"=w4338) -> ()  [unwired: 2 in, 2 out]
                }
                frame 36 {
                  n3361 = Match Pattern(string=w4339, regular expression=",") -> (before substring=→"bs":string, after substring=→"as":string)  [unwired: 1 in, 2 out]
                  n3362 = property on="Rh After" class="DigNum (strict)"("Caption.Text"=w4339) -> ()  [unwired: 2 in, 2 out]
                }
                frame 37 {
                  n3363 = Match Pattern(string=w4348, regular expression=",") -> (before substring=w4347:string, after substring=w4346:string)  [unwired: 1 in, 2 out]
                  "bs" <- w4347
                  "as" <- w4346
                  n3364 = Concatenate Strings(w4347, w4346) -> (w4343:string)
                  n3365 = property on="Humidity before test 2" class="DigNum (strict)"("Caption.Text"=w4343) -> ()  [unwired: 2 in, 2 out]
                  n3366 = property on="Humidity before test" class="DigNum (strict)"("Caption.Text"=w4343) -> ()  [unwired: 2 in, 2 out]
                  n3367 = Concatenate Strings(w4343, "=" ("string")) -> (w4344:string)
                  n3368 = local write "S 38"(w4344) -> ()
                }
                frame 38 {
                  n3369 = Match Pattern(string=w4355, regular expression=",") -> (before substring=w4354:string, after substring=w4353:string)  [unwired: 1 in, 2 out]
                  "bs" <- w4354
                  "as" <- w4353
                  n3370 = Concatenate Strings(w4354, w4353) -> (w4350:string)
                  n3371 = property on="Humidity after test 2" class="DigNum (strict)"("Caption.Text"=w4350) -> ()  [unwired: 2 in, 2 out]
                  n3372 = Concatenate Strings(w4350, "=" ("string")) -> (w4352:string)
                  n3373 = property on="Humidity after test" class="DigNum (strict)"("Caption.Text"=w4350) -> ()  [unwired: 2 in, 2 out]
                  n3374 = local write "S 39"(w4352) -> ()
                }
                frame 39 {
                  n3375 = Match Pattern(string=w4362, regular expression=",") -> (before substring=w4361:string, after substring=w4360:string)  [unwired: 1 in, 2 out]
                  "bs" <- w4361
                  "as" <- w4360
                  n3376 = Concatenate Strings(w4361, w4360) -> (w4357:string)
                  n3377 = property on="Temperature before test 2" class="DigNum (strict)"("Caption.Text"=w4357) -> ()  [unwired: 2 in, 2 out]
                  n3378 = property on="Temperature before test" class="DigNum (strict)"("Caption.Text"=w4357) -> ()  [unwired: 2 in, 2 out]
                  n3379 = Concatenate Strings(w4357, "=" ("string")) -> (→"String 34":string)
                }
                frame 40 {
                  n3380 = Match Pattern(string=w4369, regular expression=",") -> (before substring=w4368:string, after substring=w4367:string)  [unwired: 1 in, 2 out]
                  "bs" <- w4368
                  "as" <- w4367
                  n3381 = Concatenate Strings(w4368, w4367) -> (w4364:string)
                  n3382 = property on="Temperature after test 2" class="DigNum (strict)"("Caption.Text"=w4364) -> ()  [unwired: 2 in, 2 out]
                  n3383 = Concatenate Strings(w4364, "=" ("string")) -> (→"String 35":string)
                  n3384 = property on="Temperature after test" class="DigNum (strict)"("Caption.Text"=w4364) -> ()  [unwired: 2 in, 2 out]
                }
                frame 41 {
                  n3385 = property on="AVP" class="DigNum (strict)"("Caption.Text"=w4373) -> ()  [unwired: 2 in, 2 out]
                  n3386 = property on="AVP 2" class="DigNum (strict)"("Caption.Text"=w4373) -> ()  [unwired: 2 in, 2 out]
                  n3387 = Concatenate Strings(w4373, "=" ("string")) -> (→"String 36":string)
                }
                frame 42 {
                  n3388 = property on="MWSD" class="DigNum (strict)"("Caption.Text"=w4376) -> ()  [unwired: 2 in, 2 out]
                  n3389 = property on="MWSD 2" class="DigNum (strict)"("Caption.Text"=w4376) -> ()  [unwired: 2 in, 2 out]
                  n3390 = Concatenate Strings(w4376, "=" ("string")) -> (→"String 37":string)
                }
                frame 43 {
                  n3391 = property on="HCF 2" class="DigNum (strict)"("Caption.Text"=w4379) -> ()  [unwired: 2 in, 2 out]
                  n3392 = property on="HCF" class="DigNum (strict)"("Caption.Text"=w4379) -> ()  [unwired: 2 in, 2 out]
                  n3393 = Concatenate Strings(w4379, "=" ("string")) -> (→"String 38":string)
                }
                frame 44 {
                  n3394 = Concatenate Strings(w4381, "=" ("string")) -> (→"String 39":string)
                  n3395 = property on="WS1.4 2" class="DigNum (strict)"("Caption.Text"=w4381) -> ()  [unwired: 2 in, 2 out]
                  n3396 = property on="WS1.4" class="DigNum (strict)"("Caption.Text"=w4381) -> ()  [unwired: 2 in, 2 out]
                }
                frame 45 {
                  n3397 = property on="Save Results" class="Bool (strict)"("Boolean Text.Text"=w4383) -> ()  [unwired: 2 in, 2 out]
                }
                frame 46 {
                  n3398 = local write "S 47"(w4384) -> ()
                }
                frame 47 {
                  n3399 = local write "S 48"(w4385) -> ()
                }
                frame 48 {
                  n3400 = local write "S 49"(w4386) -> ()
                }
                frame 49 {
                  n3401 = local write "S 50"(w4387) -> ()
                }
                frame 50 {
                  n3402 = local write "S 51"(w4388) -> ()
                }
                frame 51 {
                  n3403 = local write "S 52"(w4389) -> ()
                }
                frame 52 {
                  n3404 = local write "S 53"(w4390) -> ()
                }
                frame 53 {
                  n3405 = local write "S 54"(w4391) -> ()
                }
                frame 54 {
                  n3406 = local write "S 55"(w4392) -> ()
                }
                frame 55 {
                  n3407 = local write "S 56"(w4393) -> ()
                }
                frame 56 {
                  n3408 = local write "S 57"(w4394) -> ()
                }
                frame 57 {
                  n3409 = local write "S 58"(w4395) -> ()
                }
                frame 58 {
                  n3410 = local write "S 59"(w4396) -> ()
                }
                frame 59 {
                  n3411 = local write "S 60"(w4397) -> ()
                }
                frame 60 {
                  n3412 = local write "S 62"(w4398) -> ()
                }
                frame 61 {
                  n3413 = local write "S 63"(w4399) -> ()
                }
                frame 62 {
                  n3414 = local write "S 64"(w4400) -> ()
                }
                frame 63 {
                  n3415 = local write "S 65"(w4401) -> ()
                }
                frame 64 {
                  n3416 = local write "S 66"(w4402) -> ()
                }
                frame 65 {
                  n3417 = local write "S 67"(w4403) -> ()
                }
                frame 66 {
                  n3418 = local write "S 68"(w4404) -> ()
                }
                frame 67 {
                  n3419 = local write "S 69"(w4405) -> ()
                }
                frame 68 {
                  n3420 = local write "S 70"(w4406) -> ()
                }
                frame 69 {
                  n3421 = local write "S 71"(w4407) -> ()
                }
                frame 70 {
                  n3422 = local write "S 72"(w4408) -> ()
                }
                frame 71 {
                  n3423 = local write "S 73"(w4409) -> ()
                }
                frame 72 {
                  n3424 = local write "S 74"(w4410) -> ()
                }
                frame 73 {
                  n3425 = local write "S 75"(w4411) -> ()
                }
                frame 74 {
                  n3426 = local write "S 76"(w4412) -> ()
                }
                frame 75 {
                  n3427 = local write "S 77"(w4413) -> ()
                }
                frame 76 {
                  n3428 = local write "S 78"(w4414) -> ()
                }
                frame 77 {
                  n3429 = local write "S 79"(w4415) -> ()
                }
                frame 79 {
                  n3430 = property on="Sample Temperature ( °C )" class="XYGraph (strict)"("Y Scale.Name Label.Text"=w4416) -> ()  [unwired: 2 in, 2 out]
                }
                frame 80 {
                  n3431 = local write "S 81"(w4417) -> ()
                  n3432 = property on="Humidity ( %RH )" class="XYGraph (strict)"("Y Scale.Name Label.Text"=w4417) -> ()  [unwired: 2 in, 2 out]
                }
                frame 78 {
                  n3433 = property on="Air Temperature  ( °C )" class="XYGraph (strict)"("X Scale.Name Label.Text"=w4418) -> ()  [unwired: 2 in, 2 out]
                  n3434 = property on="Humidity ( %RH )" class="XYGraph (strict)"("X Scale.Name Label.Text"=w4418) -> ()  [unwired: 2 in, 2 out]
                  n3435 = property on="Sample Temperature ( °C )" class="XYGraph (strict)"("X Scale.Name Label.Text"=w4418) -> ()  [unwired: 2 in, 2 out]
                  n3436 = property on="Coefficient Of Friction" class="XYGraph (strict)"("X Scale.Name Label.Text"=w4418) -> ()  [unwired: 2 in, 2 out]
                }
                frame 81 {
                  n3437 = property on="Air Temperature  ( °C )" class="XYGraph (strict)"("Y Scale.Name Label.Text"=w4419) -> ()  [unwired: 2 in, 2 out]
                }
                frame 82 {
                  n3438 = local write "S 84"(w4420) -> ()
                }
                frame 83 {
                  n3439 = local write "S 85"(w4421) -> ()
                }
                frame 84 {
                  n3440 = local write "S 86"(w4422) -> ()
                }
                frame 85 {
                  n3441 = local write "S 87"(w4423) -> ()
                }
                frame 86 {
                  n3442 = local write "S 88"(w4424) -> ()
                }
                frame 87 {
                }
                frame 88 {
                  n3443 = local write "S 90"(w4426) -> ()
                }
                frame 89 {
                  n3444 = local write "S 91"(w4427) -> ()
                }
                frame 90 {
                  n3445 = local write "S 92"(w4428) -> ()
                }
                frame 91 {
                  n3446 = local write "S 93"(w4429) -> ()
                }
                frame 92 {
                  n3447 = local write "S 94"(w4430) -> ()
                }
                frame 93 {
                  n3448 = local write "S 95"(w4431) -> ()
                }
                frame 94 {
                  n3449 = local write "S 96"(w4432) -> ()
                }
                frame 95 {
                  n3450 = local write "S 97"(w4433) -> ()
                }
                frame 96 {
                  n3451 = local write "S 98"(w4434) -> ()
                }
                frame 97 {
                  n3452 = local write "S 99"(w4435) -> ()
                }
                frame 98 {
                  n3453 = local write "S 100"(w4436) -> ()
                }
                frame 99 {
                  n3454 = local write "S 101"(w4437) -> ()
                }
                frame 100 {
                  n3455 = local write "S 102"(w4438) -> ()
                }
                frame 101 {
                  n3456 = local write "S 103"(w4439) -> ()
                }
                frame 102 {
                  n3457 = local write "S 104"(w4440) -> ()
                }
                frame 103 {
                  n3458 = local write "S 105"(w4441) -> ()
                }
                frame 104 {
                  n3459 = local write "S 106"(w4442) -> ()
                }
                frame 105 {
                }
                frame 106 {
                  n3460 = property on="OK Button 17" class="Bool (strict)"("Boolean Text.Text"=w4443) -> ()  [unwired: 2 in, 2 out]
                }
                frame 107 {
                  n3461 = property on="OK Button 16" class="Bool (strict)"("Boolean Text.Text"=w4444) -> ()  [unwired: 2 in, 2 out]
                }
                frame 108 {
                  n3462 = property on="TITTLE" class="Str"("Caption.Text"=w4445) -> ()  [unwired: 2 in, 2 out]
                }
                frame 109 {
                  "String 30" <- w4446
                }
                frame 110 {
                  n3463 = property on="Test Date" class="Str"("Caption.Text"=w4447) -> ()  [unwired: 2 in, 2 out]
                  "String 31" <- w4447
                }
                frame 111 {
                  n3464 = property on="Sample ID" class="Str"("Caption.Text"=w4448) -> ()  [unwired: 2 in, 2 out]
                  "String 32" <- w4448
                }
                frame 112 {
                  n3465 = property on="Tested by" class="Str"("Caption.Text"=w4449) -> ()  [unwired: 2 in, 2 out]
                  "String 33" <- w4449
                }
                frame 113 {
                  n3466 = property on="System Configured Printers 2" class="Arr (strict)"("Caption.Text"=w4450) -> ()  [unwired: 2 in, 2 out]
                }
                frame 114 {
                  n3467 = property on="Selected Printer" class="Str"("Caption.Text"=w4451) -> ()  [unwired: 2 in, 2 out]
                }
                frame 115 {
                  n3468 = property on="Select Printer 3" class="DigNum (strict)"("Caption.Text"=w4452) -> ()  [unwired: 2 in, 2 out]
                }
                frame 116 {
                  n3469 = property on="Print" class="Bool (strict)"("Boolean Text.Text"=w4453) -> ()  [unwired: 2 in, 2 out]
                }
                frame 117 {
                  "String 41" <- w4454
                }
                frame 118 {
                  n3470 = property on="tested by" class="Str"("Caption.Text"=w4455) -> ()  [unwired: 2 in, 2 out]
                }
                frame 119 {
                }
                frame 120 {
                  n3471 = property on="Export" class="Bool (strict)"("Boolean Text.Text"=w4456) -> ()  [unwired: 2 in, 2 out]
                }
                frame 121 {
                  n3472 = property on="TEMP INTERCEPT:" class="DigNum (strict)"("Caption.Text"=w4457) -> ()  [unwired: 2 in, 2 out]
                }
                frame 122 {
                  n3473 = property on="AIR TEMP INTERCEPT:" class="DigNum (strict)"("Caption.Text"=w4458) -> ()  [unwired: 2 in, 2 out]
                }
                frame 123 {
                  n3474 = property on="Select File Type" class="Enum (strict)"("Caption.Text"=w4459) -> ()  [unwired: 2 in, 2 out]
                }
                frame 124 {
                  n3475 = property on="s.NO" class="Str"("Caption.Text"=w4460) -> ()  [unwired: 2 in, 2 out]
                  "String 45" <- w4460
                }
                frame 125 {
                  n3476 = property on="trip1 8" class="Bool (strict)"("Boolean Text.Text"=w4461) -> ()  [unwired: 2 in, 2 out]
                }
                frame 126, Default {
                }
              }
            }
          }
          frame #1 {
            w4469 = TRUE ("Visible")
            n3477 = local read "S 91"() -> (w4486:string)
            n3478 = local read "S 90"() -> (w4485:string)
            n3479 = local read "S 88"() -> (w4484:string)
